vi "4_ВПСравнениеЧисел.vi"() -> ()   [LabVIEW 2016]
panel:
  out "Equal?":bool
  in  "Numeric 2":dbl
  in  "Numeric":dbl
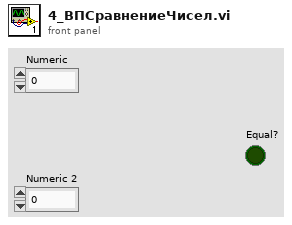
[diagram p1: front panel]
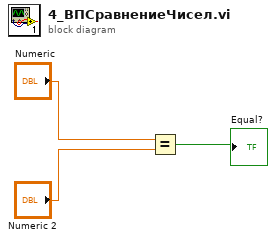
[diagram p0: block diagram]
diagram:
  n1 = Equal?(x="Numeric", y="Numeric 2") -> (x = y?=→"Equal?":bool)
